vi "get current filter.vi"(8 "error in (no error)":errorcluster, 11 "alias-tree in":refnum<class "alias-tree.lvclass">) -> (0 "error out":errorcluster, 2 "display filter":refnum<k24>, 3 "alias-tree out":refnum<class "alias-tree.lvclass">)   [LabVIEW 2017, in "vs-tree-utility.lvlib" / "alias-tree.lvclass"]
uses:
  alias-tree.lvclass
  NationalInstruments.VeriStand.SystemStorage
  NationalInstruments.VeriStand.SystemStorageUI
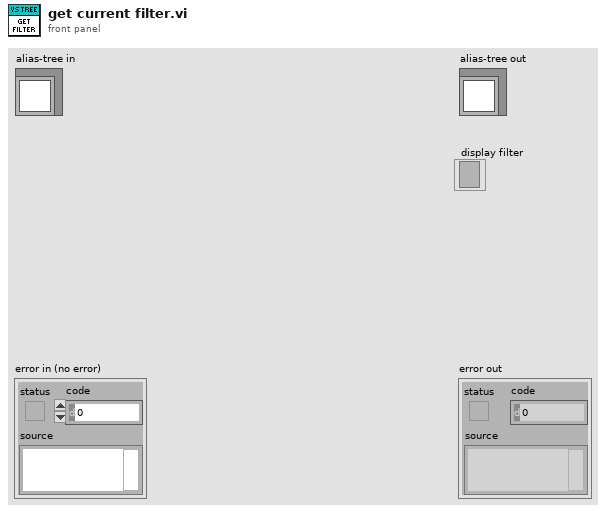
[diagram p1: front panel]
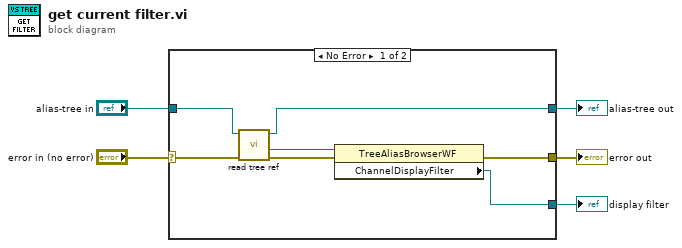
[diagram p0: block diagram]
diagram:
  n1 = case shown="No Error" "error in (no error)" {
    selector: "error in (no error)" -> [w12 w14]
    tunnel: [w8 w14] -> w4
    tunnel: [w9 w13] -> w2
    tunnel: "alias-tree in" -> [w10 w13]
    tunnel: [w6 _] -> w1
    frame No Error {
      n2 = call-dynamic "read tree ref.vi"("error in (no error)"=w12, "alias-tree in"=w10) -> ("error out"=w11:errorcluster, "tree ref"=w7:refnum<k24>, "alias-tree out"=w9:refnum<class "alias-tree.lvclass">)  [unwired: 7 in]
      n3 = property class="TreeAliasBrowserWF"(reference=w7, error in=w11) -> (error out=w8:errorcluster, "ChannelDisplayFilter"=w6:refnum<k24>)  [unwired: 1 out]
    }
    frame Error {
    }
  }
  "error out" <- w4
  "alias-tree out" <- w2
  "display filter" <- w1
